vi "Ubatt.vi"() -> ()   [LabVIEW 2020]
panel:
  out "Ubatt":dbl
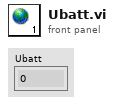
[diagram p1: front panel]
diagram:
